vi "Front Panel Defer Update.vi"(6 "Defer Panel Updates(False)":bool, 8 "error in (no error)":errorcluster, 11 "This VI":refnum<vi>) -> (0 "error out":errorcluster, 3 "This VI Out":refnum<vi>)   [LabVIEW 2015]
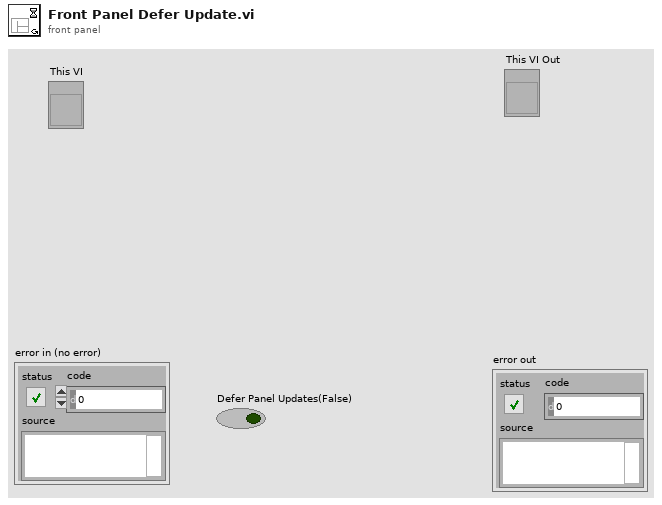
[diagram p1: front panel]
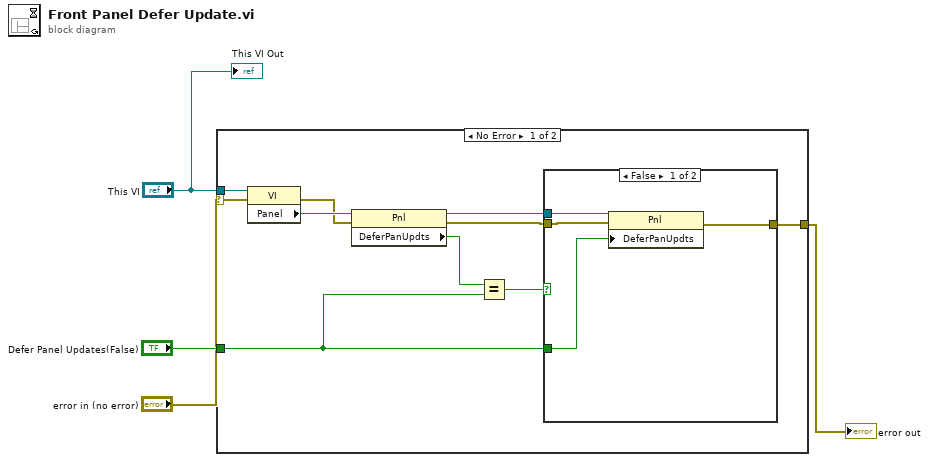
[diagram p0: block diagram]
diagram:
  n1 = case shown="No Error" "error in (no error)" {
    selector: "error in (no error)" -> [w6 w20]
    tunnel: "This VI" -> [w14 _]
    tunnel: "Defer Panel Updates(False)" -> [w10 _]
    tunnel: [w5 w20] -> w1
    frame No Error {
      n2 = property class="VI"(reference=w14, error in=w6) -> (error out=w7:errorcluster, "Panel"=w13:refnum<vi>)  [unwired: 1 out]
      n3 = property class="Pnl"(reference=w13, error in=w7) -> (reference out=w9:refnum<vi>, error out=w8:errorcluster, "DeferPanUpdts"=w12:bool)
      n4 = Equal?(x=w12, y=w10) -> (x = y?=w11:bool)
      n5 = case shown="False" w11 {
        tunnel: w10 -> [w17 _]
        tunnel: w9 -> [w18 _]
        tunnel: w8 -> [w16 w19]
        tunnel: [w15 w19] -> w5
        frame False {
          n6 = property class="Pnl"(reference=w18, error in=w16, "DeferPanUpdts"=w17) -> (error out=w15:errorcluster)  [unwired: 1 out]
        }
        frame True {
        }
      }
    }
    frame Error {
    }
  }
  "error out" <- w1
  "This VI Out" <- "This VI"
